vi "Read Lock-in driver.vi"(8 "error in (no error)":errorcluster, 11 "Lock-in in":refnum<class "Lock-in.lvclass">) -> (0 "error out":errorcluster, 2 "Lock-in Driver.lvclass":refnum<class "Lock-in Driver.lvclass">, 3 "Lock-in out":refnum<class "Lock-in.lvclass">)   [LabVIEW 2016, in "Lock-in.lvclass"]
uses:
  Lock-in.lvclass
  D:/github/Measure_core/Instrument Recorders/Instrument Recorder/Instrument Recorder.lvclass
  NHMFL_Core/Libraries/Instruments/Instrument Driver/Lock-in Driver/Lock-in Driver.lvclass
  Measure_core/Instrument Recorders/Instrument Recorder/Instrument Recorder.lvclass/Instrument Recorder.ctl
  Measure_core/Instrument Recorders/Instrument Recorder/Read Instrument driver.vi
  NHMFL_Core/Libraries/Instruments/Instrument Driver/Instrument Driver.lvclass
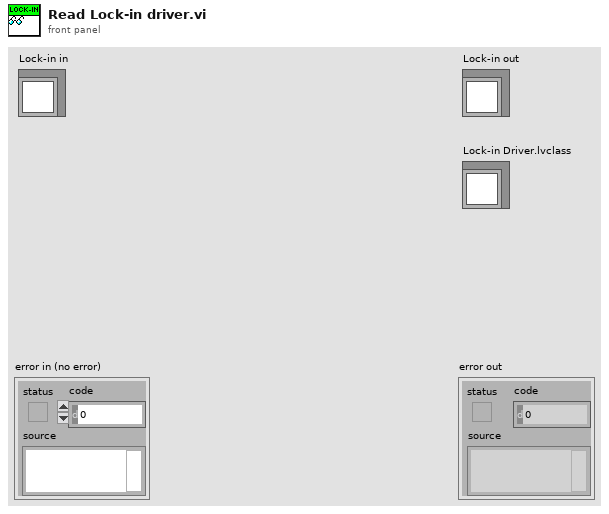
[diagram p1: front panel]
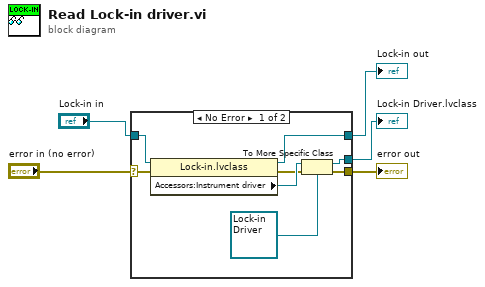
[diagram p0: block diagram]
diagram:
  n1 = case shown="No Error" "error in (no error)" {
    selector: "error in (no error)" -> [w7 w14]
    tunnel: [w11 w14] -> w4
    tunnel: [w12 w15] -> w2
    tunnel: "Lock-in in" -> [w13 w15]
    tunnel: [w6 _] -> w1
    frame No Error {
      n2 = property class="Lock-in.lvclass"(reference=w13, error in=w7) -> (reference out=w12:refnum<class "Lock-in.lvclass">, error out=w8:errorcluster, "Accessors:Instrument driver"=w9:refnum<class "Instrument Driver.lvclass">)
      n3 = To More Specific Class(target class=refnum<class "Lock-in Driver.lvclass"> refnum ("Lock-in Driver.lvclass"), reference=w9, error in=w8) -> (specific class reference=w6:refnum<class "Lock-in Driver.lvclass">, error out=w11:errorcluster)
    }
    frame Error {
    }
  }
  "error out" <- w4
  "Lock-in out" <- w2
  "Lock-in Driver.lvclass" <- w1
